vi "test.vi"() -> ()   [LabVIEW 2015]
panel:
  out "TagÉlément":string
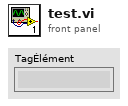
[diagram p1: front panel]
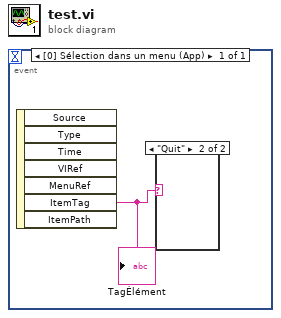
[diagram p0: block diagram]
diagram:
  n1 = event shown="[0] Sélection dans un menu (App)" {
    selector: _ -> [_]
    dyn-events: _ -> [_]
    timeout: _ -> [_]
    event Menu Selection (App) {
      n2 = event-data() -> ("ItemTag"=w1:string)  [unwired: 1 in, 6 out]
      "TagÉlément" <- w1
      n3 = case shown="\"Quit\"" w1 {
        frame "Faux", Default {
        }
        frame "Quit" {
        }
      }
    }
  }
